vi "StateGlobals.vi"() -> ()   [LabVIEW 2015]
panel:
  in  "Acquire Start Time":dbl
  out "Acquire Counter":i32
  in  "Number of Points to Acquire":i32
  out "Save Counter":i32
  in  "Experiment State":T1
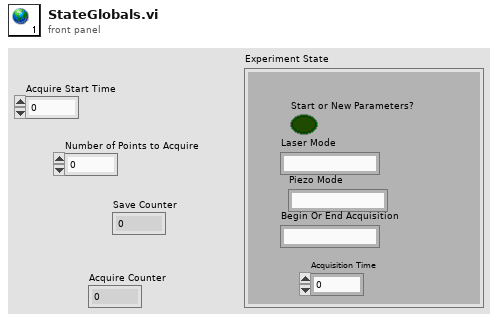
[diagram p1: front panel]
types:
  T1 = cluster{"Start or New Parameters?":bool, "Laser Mode":string, "Piezo Mode":string, "Begin Or End Acquisition":string, "Acquisition Time":dbl}
diagram:
